vi "Processamento_0323.vi"() -> ()   [LabVIEW 2017]
uses:
  <vilib>/userdefined/High Color/IMAQdx.ctl
  <vilib>/vision/driver/IMAQdx.llb/IMAQdx Acquisition Mode.ctl
  <vilib>/vision/driver/IMAQdx.llb/IMAQdx Buffer Number Mode.ctl
  <vilib>/vision/Measure.llb/Edge Options.ctl
  <vilib>/vision/Measure.llb/Edge Polarity.ctl
  <vilib>/vision/Measure.llb/Straight Edge Options.ctl
  <vilib>/vision/Measure.llb/Straight Edge Process.ctl
  <vilib>/vision/Classification.llb/IMAQ Classifier Read Options.ctl
  <vilib>/vision/driver/NI_Vision_Acquisition_Software.lvlib
  <vilib>/vision/NI_Vision_Development_Module.lvlib
  <resource>/objmgr/IMAQImage.rc
panel:
  out "Array":T1(array[cluster])
  out "error out 2":errorcluster
  out "error out":errorcluster
  in  "Classificador de cor":path
  out "Imagem Processada":T2(plugin-control)
  in  "Stop Button":bool
  out "Imagem Original":T2(plugin-control)
  in  "Session In":T3="cam1"
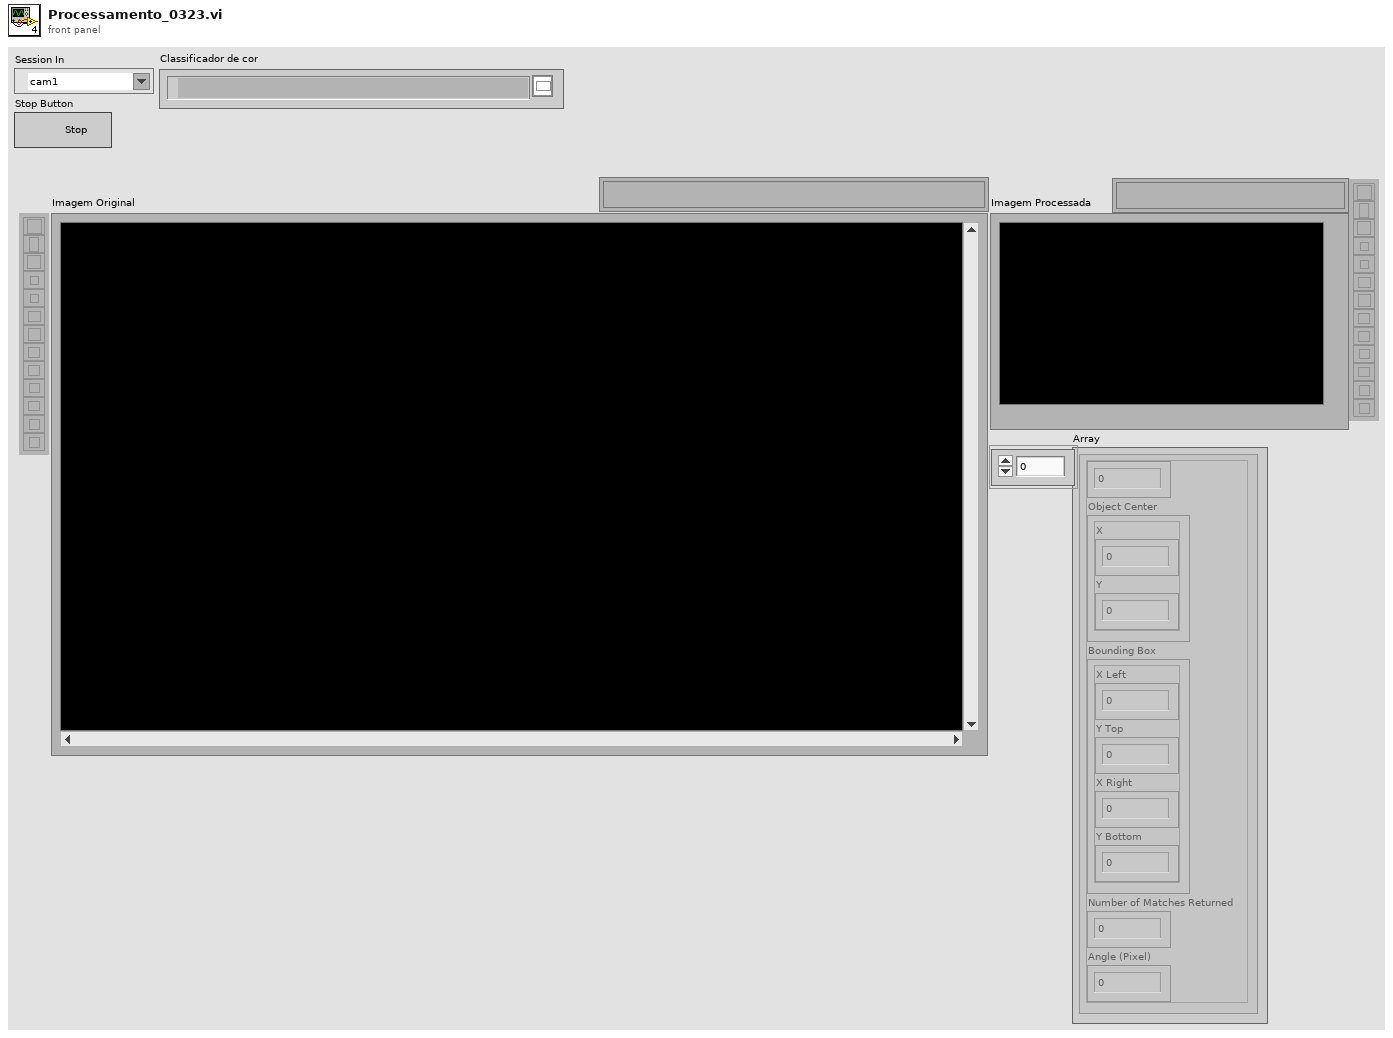
[diagram p1: front panel]
types:
  T1 = cluster{"Numeric Control":i32, "Object Center":cluster{"X":sgl, "Y":sgl}, "Bounding Box":cluster{"X Left":i32, "Y Top":i32, "X Right":i32, "Y Bottom":i32}, "Number of Matches Returned":i32, "Angle (Pixel)":dbl}[]
  T2 = typedef "IMAQ Image.ctl" = refnum<image>
  T3 = typedef "IMAQdx.ctl" = refnum<k21>
  T4 = typedef "Image Type" = u32
  T5 = typedef "NI_Vision_Acquisition_Software.lvlib/IMAQdx Acquisition Mode.ctl" = enum32{"One Shot", "Continuous"}
  T6 = cluster{"Objects":u16, "Threshold":i32, "Reject Border":bool, "Fill Holes":bool, "Min Object Size":bool, "Min Size":i32, "Max Object Size":bool, "Max Size":i32, "Show Search Area":bool, "Show Center":bool, "Show Bounding Box":bool}
  T7 = enum32{"AutoM", "Close", "Dilate", "Erode", "Gradient", "Gradient out", "Gradient in", "Hit miss", "Open", "PClose", "POpen", "Thick", "Thin"}
  T8 = typedef "Edge Options.ctl" = cluster{"Edge Polarity":T9, "Kernel Size":u32, "Width":u32, "Minimum Edge Strength":sgl, "Interpolation Type":enum32{"Zero Order", "Bilinear", "Quadratic", "Cubic", "Bilinear Fixed"}, "Data Processing Method":enum32{"Average", "Median"}}
  T9 = typedef "Edge Polarity.ctl" = u32
  T10 = cluster{"Search Direction":u32, "Edge Options":T8, "Show Search Area":bool, "Show Search Lines":bool, "Show Edges Found":bool, "Show Result":bool, "Search Area Color":u32, "Search Lines Color":u32, "Edge Locations Color":u32, "Result Color":u32, "Overlay Group Name":string}
  T11 = typedef "NI_Vision_Acquisition_Software.lvlib/IMAQdx Buffer Number Mode.ctl" = enum32{"Next", "Last", "Buffer Number", "Every", "Last New"}
  T12 = typedef "Straight Edge Options.ctl" = cluster{"Number of Lines":i32, "Type":T13, "Min. Score":dbl, "Max. Score":dbl, "Orientation":dbl, "Angle Range":dbl, "Angle Tolerance":dbl, "Step Size":u32, "Min. SNR (db)":dbl, "Min. Points (%)":dbl, "Hough Iterations":i32}
  T13 = typedef "Straight Edge Process.ctl" = enum32{"First Edge Rake", "Best Edge Rake", "Hough Edge Rake", "First Edge Projection", "Best Edge Projection"}
  T14 = cluster{"Desired Font (Application)":enum16{"User-specified Font", "Application Font", "System Font", "Dialog Font"}, "[User-specified Font]":cluster{"Font Name":string, "Size":i16, "Strikeout?":bool, "Italic?":bool, "Underline?":bool, "Outline?":bool, "Shadow?":bool, "Bold?":bool, "Rotation Angle":dbl}, "Horizontal Alignment":i16, "Vertical Alignment":i16}
  T15 = cluster{"Extraction Mode":u32, "Edge Threshold":i32, "Edge Filter Size":u32, "Min Length":i32, "Row Search Step Size":i32, "Col Search Step Size":i32, "Max Endpoint Gap":i32, "Closed":bool, "Subpixel":bool}
  T16 = cluster{"Rotation":bool, "Scale":bool, "Occlusion":bool, "Range Settings":cluster{"Match Constraints":u32, "Min":dbl, "Max":dbl}[]}
  T17 = cluster{"element":dbl, "y":i32, "x":i32, "element":dbl, "element":dbl}
  T18 = typedef "ROI Descriptor" = cluster{"Global Rectangle":i32[], "Contours":cluster{"ID":enum32{"External", "Internal"}, "Type":u32, "Coordinates":i32[]}[]}
  T19 = cluster{"Point1 (Pixels)":cluster{"X":sgl, "Y":sgl}, "Point2 (Pixels)":cluster{"X":sgl, "Y":sgl}, "Point1 (Real-World)":cluster{"X":sgl, "Y":sgl}, "Point2 (Real-World)":cluster{"X":sgl, "Y":sgl}, "Angle (Pixel)":dbl, "Angle (Real-World)":dbl, "Score":dbl, "Straightness":dbl, "Average SNR (db)":dbl, "Calibration Valid":bool}[]
  T20 = cluster{"Point1 (Pixels)":cluster{"X":sgl, "Y":sgl}, "Point2 (Pixels)":cluster{"X":sgl, "Y":sgl}, "Point1 (Real-World)":cluster{"X":sgl, "Y":sgl}, "Point2 (Real-World)":cluster{"X":sgl, "Y":sgl}, "Angle (Pixel)":dbl, "Angle (Real-World)":dbl, "Score":dbl, "Straightness":dbl, "Average SNR (db)":dbl, "Calibration Valid":bool}
  T21 = cluster{"element":dbl, sgl, "x":i32, sgl, "element":dbl}
  T22 = cluster{"Object Center":cluster{"X":sgl, "Y":sgl}, "Bounding Box":cluster{"X Left":i32, "Y Top":i32, "X Right":i32, "Y Bottom":i32}, "Area":sgl, "Orientation":sgl, "Aspect Ratio":sgl, "Nb Holes":i32}[]
  T23 = cluster{"X Left":i32, "Y Top":i32, "X Right":i32, "Y Bottom":i32}
  T24 = typedef "IMAQ Classifier Read Options.ctl" = i32
  T25 = typedef "IMAQ Classifier Session.ctl" = refnum<k1>
  T26 = cluster{i32, "Object Center":cluster{"X":sgl, "Y":sgl}, "Bounding Box":cluster{"X Left":i32, "Y Top":i32, "X Right":i32, "Y Bottom":i32}, "Number of Matches Returned":i32, "Angle (Pixel)":dbl}
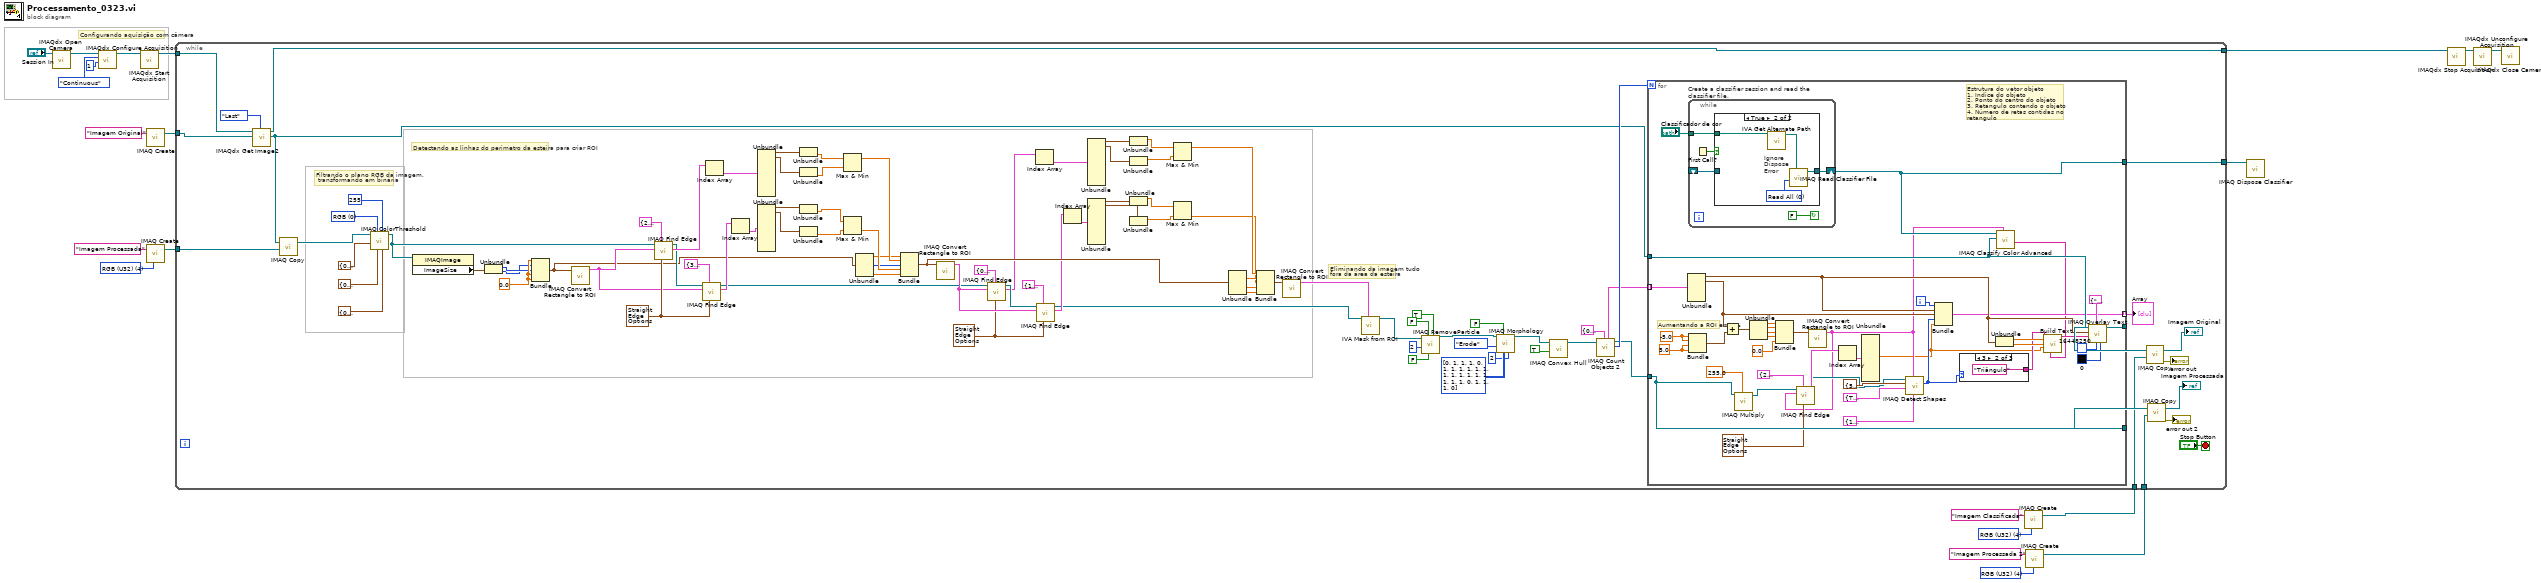
[diagram p0: block diagram]
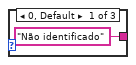
[diagram p2: hidden frame]
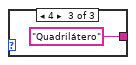
[diagram p3: hidden frame]
diagram:
  w3 = T4 4 items=["Grayscale (U8)", "Grayscale (I16)", "Grayscale (SGL)", "Complex (CSG)", "RGB (U32)", "HSL (U32)", "RGB (U64)", "Grayscale (U16)"] ("Image Type")
  w6 = T4 4 items=["Grayscale (U8)", "Grayscale (I16)", "Grayscale (SGL)", "Complex (CSG)", "RGB (U32)", "HSL (U32)", "RGB (U64)", "Grayscale (U16)"] ("Image Type")
  w10 = T4 4 items=["Grayscale (U8)", "Grayscale (I16)", "Grayscale (SGL)", "Complex (CSG)", "RGB (U32)", "HSL (U32)", "RGB (U64)", "Grayscale (U16)"] ("Image Type")
  # "Configurando aquisição com câmera"
  n1 = call <vilib>:"IMAQdx Open Camera.vi"("Session In"="Session In") -> ("Session Out"=w21:T3)  [unwired: 9 in, 1 out]
  n2 = call <vilib>:"IMAQdx Configure Acquisition.vi"("Number of Buffers"=u32 1, "Continuous?"=IMAQdx_Acquisition_Mode."Continuous", "Session In"=w21) -> ("Session Out"=w20:T3)  [unwired: 7 in, 1 out]
  n3 = call <vilib>:"IMAQdx Start Acquisition.vi"("Session In"=w20) -> ("Session Out"=w9:T3)  [unwired: 9 in, 1 out]
  n4 = call "IMAQ Create"("Image Name"="Imagem Processada", "Image Type"=w10) -> ("New Image"=w11:T2)  [unwired: 3 in, 1 out]
  n5 = call "IMAQ Create"("Image Name"="Imagem Original") -> ("New Image"=w15:T2)  [unwired: 4 in, 1 out]
  n6 = call "IMAQ Create"("Image Name"="Imagem Classificada", "Image Type"=w3) -> ("New Image"=w2:T2)  [unwired: 3 in, 1 out]
  n7 = call "IMAQ Create"("Image Name"="Imagem Processada 2", "Image Type"=w6) -> ("New Image"=w5:T2)  [unwired: 3 in, 1 out]
  n8 = while {
    tunnel: w15 -> [w116]
    tunnel: w11 -> [w113]
    tunnel: w9 -> [w37]
    tunnel: [w36] -> w8
    tunnel: w5 -> [w30]
    tunnel: w2 -> [w27]
    tunnel: [w25] -> w1
    stop <- "Stop Button" stop-if-true
    w74 = T12 {"Number of Lines"=1, "Type"=enum."First Edge Rake", "Min. Score"=10.0, "Max. Score"=1000.0, "Orientation"=0.0, "Angle Range"=45.0, "Angle Tolerance"=1.0, "Step Size"=32, "Min. SNR (db)"=0.0, "Min. Points (%)"=25.0, "Hough Iterations"=5} ("Fit Options")
    w99 = T12 {"Number of Lines"=1, "Type"=enum."First Edge Rake", "Min. Score"=10.0, "Max. Score"=1000.0, "Orientation"=0.0, "Angle Range"=45.0, "Angle Tolerance"=1.0, "Step Size"=32, "Min. SNR (db)"=0.0, "Min. Points (%)"=25.0, "Hough Iterations"=5} ("Fit Options")
    w105 = 0.0 ("element")
    w108 = u16 0 items=["RGB", "HSL", "HSV", "HSI"] ("Color Mode")
    # "Eliminando da imagem tudo\nfora da área da esteira"
    # "Detectando as linhas do perimetro da esteira para criar ROI"
    # "Filtrando o plano RGB da imagem,\n transformando em binária"
    n9 = call <vilib>:"IMAQdx Get Image2.vi"("Buffer Number Mode (Next)"=IMAQdx_Buffer_Number_Mode."Last", "Image In"=w116, "Session In"=w37) -> ("Image Out"=w33:T2, "Session Out"=w36:T3)  [unwired: 5 in, 2 out]
    n10 = call "IMAQ Copy"("Image Dst"=w113, "Image Src"=w33) -> ("Image Dst Out"=w107:T2)  [unwired: 4 in, 1 out]
    n11 = call "IMAQ ColorThreshold"("Blue or Luma or Val or Inten Range"=cluster{"Lower value":i32, "Upper value":i32} {"Lower value"=0, "Upper value"=170}, "Replace Value"=255, "Green or Sat Range"=cluster{"Lower value":i32, "Upper value":i32} {"Lower value"=0, "Upper value"=255}, "Color Mode"=w108, "Red or Hue Range"=cluster{"Lower value":i32, "Upper value":i32} {"Lower value"=0, "Upper value"=255}, "Image Src"=w107) -> ("Image Dst Out"=w103:T2)  [unwired: 2 in, 3 out]
    n12 = property class="IMAQImage"(reference=w103) -> ("ImageSize"=w106:cluster{"x":i32, "y":i32})  [unwired: 1 in, 2 out]
    n13 = Unbundle(w106) -> ("x"=w102:i32, "y"=w101:i32)
    n14 = Bundle("element"=w105, "y"=w101, "x"=w102, "element"=w105, "element"=w105) -> (w72:T17)  [unwired: 1 in]
    n15 = call "IMAQ Convert Rectangle to ROI"("Rectangle"=w72) -> ("ROI Descriptor"=w98:T18)  [unwired: 8 in, 1 out]
    n16 = call "IMAQ Find Edge"("Line Fit Options"=w99, "Options"=T10 {"Search Direction"=2, "Edge Options"={"Edge Polarity"=2, "Kernel Size"=3, "Width"=1, "Minimum Edge Strength"=80.0, "Interpolation Type"=enum."Bilinear Fixed", "Data Processing Method"=enum."Average"}, "Show Search Area"=FALSE, "Show Search Lines"=FALSE, "Show Edges Found"=FALSE, "Show Result"=FALSE, "Search Area Color"=65280, "Search Lines Color"=255, "Edge Locations Color"=16776960, "Result Color"=16711680, "Overlay Group Name"=""}, "ROI Descriptor"=w98, "Image"=w103) -> ("Straight Edges"=w100:T19, "Image Out"=w97:T2)  [unwired: 2 in, 4 out]
    n17 = call "IMAQ Find Edge"("Line Fit Options"=w99, "Options"=T10 {"Search Direction"=3, "Edge Options"={"Edge Polarity"=2, "Kernel Size"=3, "Width"=1, "Minimum Edge Strength"=80.0, "Interpolation Type"=enum."Bilinear Fixed", "Data Processing Method"=enum."Average"}, "Show Search Area"=FALSE, "Show Search Lines"=FALSE, "Show Edges Found"=FALSE, "Show Result"=FALSE, "Search Area Color"=65280, "Search Lines Color"=255, "Edge Locations Color"=16776960, "Result Color"=16711680, "Overlay Group Name"=""}, "ROI Descriptor"=w98, "Image"=w97) -> ("Straight Edges"=w95:T19, "Image Out"=w75:T2)  [unwired: 2 in, 4 out]
    n18 = Index Array(array=w100) -> (element=w94:T20)  [unwired: 1 in]
    n19 = Index Array(array=w95) -> (element=w93:T20)  [unwired: 1 in]
    n20 = Unbundle(w94) -> ("Point1 (Pixels)"=w92:cluster{"X":sgl, "Y":sgl}, "Point2 (Pixels)"=w91:cluster{"X":sgl, "Y":sgl})  [unwired: 8 out]
    n21 = Unbundle(w93) -> ("Point1 (Pixels)"=w90:cluster{"X":sgl, "Y":sgl}, "Point2 (Pixels)"=w89:cluster{"X":sgl, "Y":sgl})  [unwired: 8 out]
    n22 = Unbundle(w92) -> ("Y"=w88:sgl)  [unwired: 1 out]
    n23 = Unbundle(w91) -> ("Y"=w87:sgl)  [unwired: 1 out]
    n24 = Unbundle(w90) -> ("Y"=w86:sgl)  [unwired: 1 out]
    n25 = Unbundle(w89) -> ("Y"=w85:sgl)  [unwired: 1 out]
    n26 = Max & Min(x=w88, y=w87) -> (max(x,y)=w84:sgl)  [unwired: 1 out]
    n27 = Max & Min(x=w86, y=w85) -> (min(x,y)=w83:sgl)  [unwired: 1 out]
    n28 = Unbundle(w72) -> ("element"=w81:dbl, "x"=w82:i32, "element"=w80:dbl)  [unwired: 2 out]
    n29 = Bundle("element"=w81, w84, "x"=w82, w83, "element"=w80) -> (w70:T21)  [unwired: 1 in]
    n30 = call "IMAQ Convert Rectangle to ROI"("Rectangle"=w70) -> ("ROI Descriptor"=w77:T18)  [unwired: 8 in, 1 out]
    n31 = call "IMAQ Find Edge"("Line Fit Options"=w74, "Options"=T10 {"Search Direction"=0, "Edge Options"={"Edge Polarity"=2, "Kernel Size"=3, "Width"=1, "Minimum Edge Strength"=80.0, "Interpolation Type"=enum."Bilinear Fixed", "Data Processing Method"=enum."Average"}, "Show Search Area"=FALSE, "Show Search Lines"=FALSE, "Show Edges Found"=FALSE, "Show Result"=FALSE, "Search Area Color"=65280, "Search Lines Color"=255, "Edge Locations Color"=16776960, "Result Color"=16711680, "Overlay Group Name"=""}, "ROI Descriptor"=w77, "Image"=w75) -> ("Straight Edges"=w61:T19, "Image Out"=w76:T2)  [unwired: 2 in, 4 out]
    n32 = Index Array(array=w61) -> (element=w65:T20)  [unwired: 1 in]
    n33 = call "IMAQ Find Edge"("Line Fit Options"=w74, "Options"=T10 {"Search Direction"=1, "Edge Options"={"Edge Polarity"=2, "Kernel Size"=3, "Width"=1, "Minimum Edge Strength"=80.0, "Interpolation Type"=enum."Bilinear Fixed", "Data Processing Method"=enum."Average"}, "Show Search Area"=FALSE, "Show Search Lines"=FALSE, "Show Edges Found"=FALSE, "Show Result"=FALSE, "Search Area Color"=65280, "Search Lines Color"=255, "Edge Locations Color"=16776960, "Result Color"=16711680, "Overlay Group Name"=""}, "ROI Descriptor"=w77, "Image"=w76) -> ("Straight Edges"=w60:T19, "Image Out"=w52:T2)  [unwired: 2 in, 4 out]
    n34 = Index Array(array=w60) -> (element=w64:T20)  [unwired: 1 in]
    n35 = Unbundle(w65) -> ("Point1 (Pixels)"=w66:cluster{"X":sgl, "Y":sgl}, "Point2 (Pixels)"=w67:cluster{"X":sgl, "Y":sgl})  [unwired: 8 out]
    n36 = Unbundle(w64) -> ("Point1 (Pixels)"=w63:cluster{"X":sgl, "Y":sgl}, "Point2 (Pixels)"=w62:cluster{"X":sgl, "Y":sgl})  [unwired: 8 out]
    n37 = Unbundle(w66) -> ("X"=w57:sgl)  [unwired: 1 out]
    n38 = Unbundle(w67) -> ("X"=w56:sgl)  [unwired: 1 out]
    n39 = Unbundle(w63) -> ("X"=w55:sgl)  [unwired: 1 out]
    n40 = Unbundle(w62) -> ("X"=w54:sgl)  [unwired: 1 out]
    n41 = Max & Min(x=w57, y=w56) -> (max(x,y)=w59:sgl)  [unwired: 1 out]
    n42 = Max & Min(x=w55, y=w54) -> (min(x,y)=w58:sgl)  [unwired: 1 out]
    n43 = Unbundle(w70) -> (w69:sgl, w68:sgl, "element"=w71:dbl)  [unwired: 2 out]
    n44 = Bundle(w59, w69, w58, w68, "element"=w71) -> (w73:cluster{sgl, sgl, sgl, sgl, "element":dbl})  [unwired: 1 in]
    n45 = call "IMAQ Convert Rectangle to ROI"("Rectangle"=w73) -> ("ROI Descriptor"=w53:T18)  [unwired: 8 in, 1 out]
    n46 = call <vilib>:"IVA Mask from ROI.vi"("ROI Descriptor"=w53, "Image Src"=w52) -> ("Image Out"=w47:T2)  [unwired: 3 in, 6 out]
    n47 = call "IMAQ RemoveParticle"("Connectivity 4/8 (8)"=TRUE, "Low Pass/High Pass (Low)"=FALSE, "Square/Hexa (Square)"=FALSE, "Number of Erosion"=2, "Image Src"=w47) -> ("Image Dst Out"=w42:T2)  [unwired: 2 in, 4 out]
    n48 = call "IMAQ Morphology"("Number of iterations (1)"=2, "Structuring Element"=i32[][] [[0, 1, 1, 1, 0], [1, 1, 1, 1, 1], [1, 1, 1, 1, 1], [1, 1, 1, 1, 1], [0, 1, 1, 1, 0]], "Square/Hexa (Square)"=FALSE, "Operation"=T7."Erode", "Image Src"=w42) -> ("Image Dst Out"=w40:T2)  [unwired: 2 in, 4 out]
    n49 = call "IMAQ Convex Hull"("Connectivity 4/8 (8)"=TRUE, "Image Src"=w40) -> ("Image Dst Out"=w39:T2)  [unwired: 2 in, 7 out]
    n50 = call "IMAQ Count Objects 2"("Settings"=T6 {"Objects"=0, "Threshold"=1, "Reject Border"=FALSE, "Fill Holes"=FALSE, "Min Object Size"=TRUE, "Min Size"=400, "Max Object Size"=FALSE, "Max Size"=100, "Show Search Area"=FALSE, "Show Center"=FALSE, "Show Bounding Box"=FALSE}, "Image"=w39) -> ("Number of Objects"=w35:i32, "Image Out"=w32:T2, "Objects"=w34:T22)  [unwired: 5 in, 2 out]
    n51 = for {
      N: w35 -> [_]
      tunnel: w34 -> [w154] mode=indexing
      tunnel: w33 -> [w133]
      tunnel: w32 -> [w125]
      tunnel: [w125] -> w31
      tunnel: [w135] -> w28
      tunnel: [w130] -> w25
      tunnel: [w129] -> w22 mode=indexing
      i -> [w143]
      w153 = -5.0
      w152 = 5.0
      # "Estrutura do vetor objeto\n1. Indice do objeto\n2. Ponto do centro do objeto\n3. Retangulo contendo o objeto\n4. Número de retas contidas no retangulo"
      # "Aumentando a ROI em 5%"
      n52 = Unbundle(w154) -> ("Object Center"=w138:cluster{"X":sgl, "Y":sgl}, "Bounding Box"=w131:T23)  [unwired: 4 out]
      n53 = while "Create a classifier session and read the classifier file." {
        shift-right: [w165] -> w130
        shift-left: _ -> [w161]
        tunnel: "Classificador de cor" -> [w163]
        stop <- FALSE continue-if-true
        n54 = First Call?() -> (First Call?: T/F=w162:bool)
        n55 = case shown="True" w162 {
          tunnel: [w166 w169] -> w165
          tunnel: w163 -> [_ w168]
          tunnel: w161 -> [w166 _]
          frame False {
          }
          frame True {
            w170 = T24 0 items=["Read All", "Add Samples, Do Not Change Options", "Read Options, Do Not Add Samples"] ("Read Options")
            # "Ignore Dispose Error"
            n56 = call <vilib>:"IVA Get Alternate Path.vi"("Path In"=w168) -> ("Path Out"=w167:path)  [unwired: 10 out]
            n57 = call "IMAQ Read Classifier File"("File Path"=w167, "Read Options"=w170) -> ("Classifier Session"=w169:T25)  [unwired: 2 in, 7 out]
          }
        }
      }
      n58 = Bundle(w153, w153, w152, w152) -> (w151:cluster{dbl, dbl, dbl, dbl})  [unwired: 1 in]
      n59 = Add(x=w131, y=w151) -> (x+y=w150:cluster{dbl, dbl, dbl, dbl})
      n60 = call "IMAQ Multiply"("Image Src A"=w125, "Constant"=255.0) -> ("Image Dst Out"=w123:T2)  [unwired: 5 in, 1 out]
      n61 = Unbundle(w150) -> (w149:dbl, w148:dbl, w147:dbl, w146:dbl)
      n62 = Bundle(w149, w148, w147, w146, 0.0) -> (w144:cluster{dbl, dbl, dbl, dbl, dbl})  [unwired: 1 in]
      n63 = call "IMAQ Convert Rectangle to ROI"("Rectangle"=w144) -> ("ROI Descriptor"=w118:T18)  [unwired: 8 in, 1 out]
      n64 = call "IMAQ Find Edge"("Line Fit Options"=T12 {"Number of Lines"=1, "Type"=enum."First Edge Rake", "Min. Score"=10.0, "Max. Score"=1000.0, "Orientation"=0.0, "Angle Range"=180.0, "Angle Tolerance"=1.0, "Step Size"=32, "Min. SNR (db)"=0.0, "Min. Points (%)"=25.0, "Hough Iterations"=5} ("Fit Options"), "Options"=T10 {"Search Direction"=2, "Edge Options"={"Edge Polarity"=2, "Kernel Size"=3, "Width"=1, "Minimum Edge Strength"=80.0, "Interpolation Type"=enum."Bilinear Fixed", "Data Processing Method"=enum."Average"}, "Show Search Area"=TRUE, "Show Search Lines"=TRUE, "Show Edges Found"=TRUE, "Show Result"=TRUE, "Search Area Color"=65280, "Search Lines Color"=255, "Edge Locations Color"=16776960, "Result Color"=16711680, "Overlay Group Name"=""}, "ROI Descriptor"=w118, "Image"=w123) -> ("Straight Edges"=w120:T19, "Image Out"=w119:T2)  [unwired: 4 in, 2 out]
      n65 = Index Array(array=w120) -> (element=w126:T20)  [unwired: 1 in]
      n66 = Unbundle(w126) -> ("Angle (Pixel)"=w117:dbl)  [unwired: 9 out]
      n67 = call-poly "IMAQ Detect Shapes"("Curve Parameters"=T15 {"Extraction Mode"=1, "Edge Threshold"=1, "Edge Filter Size"=1, "Min Length"=50, "Row Search Step Size"=15, "Col Search Step Size"=15, "Max Endpoint Gap"=10, "Closed"=FALSE, "Subpixel"=FALSE}, "ROI Descriptor"=w118, "Match Options"=T16 {"Rotation"=TRUE, "Scale"=FALSE, "Occlusion"=FALSE, "Range Settings"=[{"Match Constraints"=0, "Min"=0.0, "Max"=360.0}]}, "Line Descriptor"=cluster{"Min Length":dbl, "Max Length":dbl} {"Min Length"=50.0, "Max Length"=500.0}, "Image"=w119) -> ("Number of Matches Returned"=w132:i32)  [unwired: 4 in, 2 out]
      n68 = Bundle(w143, "Object Center"=w138, "Bounding Box"=w131, "Number of Matches Returned"=w132, "Angle (Pixel)"=w117) -> (w129:T26)  [unwired: 1 in]
      n69 = case shown="3" w132 {
        tunnel: ["Não identificado" "Triângulo" "Quadrilátero"] -> w127
        frame 0, Default {
        }
        frame 3 {
        }
        frame 4 {
        }
      }
      n70 = Unbundle(w138) -> ("X"=w142:sgl, "Y"=w141:sgl)
      n71 = call "IMAQ Classify Color Advanced"("ROI Descriptor"=w118, "Image"=w133, "Classifier Session"=w130) -> ("Class"=w128:string)  [unwired: 1 in, 7 out]
      n72 = call "Build Text"("forma"=w127, "x"=w142, "y"=w141, "orientação"=w117, "cor"=w128) -> ("Result"=w139:string)  [unwired: 9 in, 1 out]
      n73 = call "IMAQ Overlay Text"("BG Color (Transparent)"=u32 0, "Text Color (black)"=u32 16448250, "Font, Size & Style"=T14 {"Desired Font (Application)"=enum."Application Font", "[User-specified Font]"={"Font Name"="", "Size"=12, "Strikeout?"=FALSE, "Italic?"=FALSE, "Underline?"=FALSE, "Outline?"=FALSE, "Shadow?"=FALSE, "Bold?"=TRUE, "Rotation Angle"=0.0}, "Horizontal Alignment"=1, "Vertical Alignment"=2}, "String"=w139, "Origin"=w138, "Image"=w133) -> ("Image Out"=w135:T2)  [unwired: 4 in, 1 out]
    }
    "Array" <- w22
    n74 = call "IMAQ Copy"("Image Dst"=w27, "Image Src"=w28) -> ("error out"=→"error out":errorcluster, "Image Dst Out"=→"Imagem Original":T2)  [unwired: 4 in]
    n75 = call "IMAQ Copy"("Image Dst"=w30, "Image Src"=w31) -> ("error out"=→"error out 2":errorcluster, "Image Dst Out"=→"Imagem Processada":T2)  [unwired: 4 in]
  }
  n76 = call "IMAQ Dispose Classifier"("Classifier Session"=w1) -> ()  [unwired: 1 in, 10 out]
  n77 = call <vilib>:"IMAQdx Stop Acquisition.vi"("Session In"=w8) -> ("Session Out"=w19:T3)  [unwired: 9 in, 1 out]
  n78 = call <vilib>:"IMAQdx Unconfigure Acquisition.vi"("Session In"=w19) -> ("Session Out"=w18:T3)  [unwired: 9 in, 1 out]
  n79 = call <vilib>:"IMAQdx Close Camera.vi"("Session In"=w18) -> ()  [unwired: 10 in, 1 out]
